vi "Calib_Change.vi"(1 "Eng Units":dbl[][](array[numeric]) format="%.2f") -> (0 "% Change":dbl format="%.4f")   [LabVIEW 2010]
uses:
  <vilib>/Analysis/NI_AALBase.lvlib
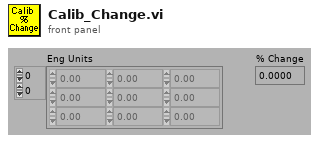
[diagram p1: front panel]
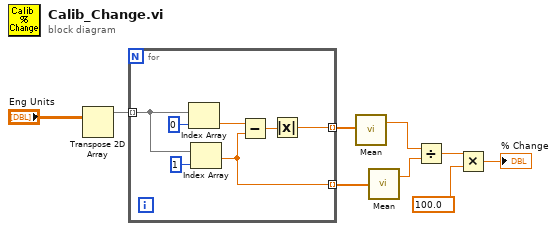
[diagram p0: block diagram]
diagram:
  n1 = Transpose 2D Array(2D array="Eng Units") -> (transposed array=w3:dbl[][])
  n2 = for {
    tunnel: w3 -> [w14] mode=indexing
    tunnel: [w12] -> w4 mode=indexing
    tunnel: [w11] -> w5 mode=indexing
    n3 = Index Array(array=w14, index=0 ("Index")) -> (element=w10:dbl)
    n4 = Index Array(array=w14, index=1 ("Index")) -> (element=w11:dbl)
    n5 = Subtract(x=w10, y=w11) -> (x-y=w13:dbl)
    n6 = Absolute Value(x=w13) -> (abs(x)=w12:dbl)
  }
  n7 = call <vilib>:"Mean.vi"("X"=w4) -> ("mean"=w7:dbl)  [unwired: 1 out]
  n8 = call <vilib>:"Mean.vi"("X"=w5) -> ("mean"=w6:dbl)  [unwired: 1 out]
  n9 = Divide(x=w7, y=w6) -> (x/y=w8:dbl)
  n10 = Multiply(x=w8, y=100.0) -> (x*y=→"% Change":dbl)
